vi "MFP assistant - Check leads connections.vi"(8 "Source":dbl[](array[numeric])=[1.0, 2.0, 3.0, 4.0, 5.0, 27.0, 28.0], 9 "Wait after changing source":dbl=5000.0, 10 "shunt resistor":dbl=100000.0 format="%#_13g", 11 "Excitation voltage":dbl=0.1) -> ()   [LabVIEW 2016]
uses:
  <userlib>/LevyLab/Lockin-Multichannel/Typedefs/AO-cluster.ctl
  <userlib>/LevyLab/Lockin-Multichannel/Typedefs/AO_Amp-array.ctl
  <userlib>/LevyLab/Lockin-Multichannel/Typedefs/AO_DC-array.ctl
  <userlib>/LevyLab/Lockin-Multichannel/Typedefs/AO_f-array.ctl
  <userlib>/LevyLab/Lockin-Multichannel/Typedefs/AO_phi-array.ctl
  <userlib>/LevyLab/Lockin-Multichannel/Typedefs/Function-array.ctl
  <userlib>/LevyLab/Lockin-Multichannel/Typedefs/Function-enum.ctl
panel:
  out "error out":errorcluster={"status"=TRUE, "code"=1000, "source"="Invoke Node in MFP assistant - Check leads connections.vi\n<APPEND>\nMethod Name: <b>Run VI</b>\n\nVI Path: <b>C:\\Program Files (x86)\\National Instruments\\LabVIEW 2016\\user.lib\\LevyLab\\Lockin-Multichannel\\Lockin-4461 -Patrick -State.vi</b>"}
  out "Drain":dbl=2.0
  out "Source":dbl=2.0
  out "2-T G":dbl=1.9062096105905893e-11 format="%#_6p"
  out "2-T G":dbl[][](array[numeric])=[[-1.000136832285521e-05, 1.2511313986118265e-10], [-4.380879926044356e-11, 1.9062096105905893e-11]] format="%#_4p"
  out "Drain":dbl[](array[numeric])=[1.0, 2.0]
  out "reference out":refnum<vi>
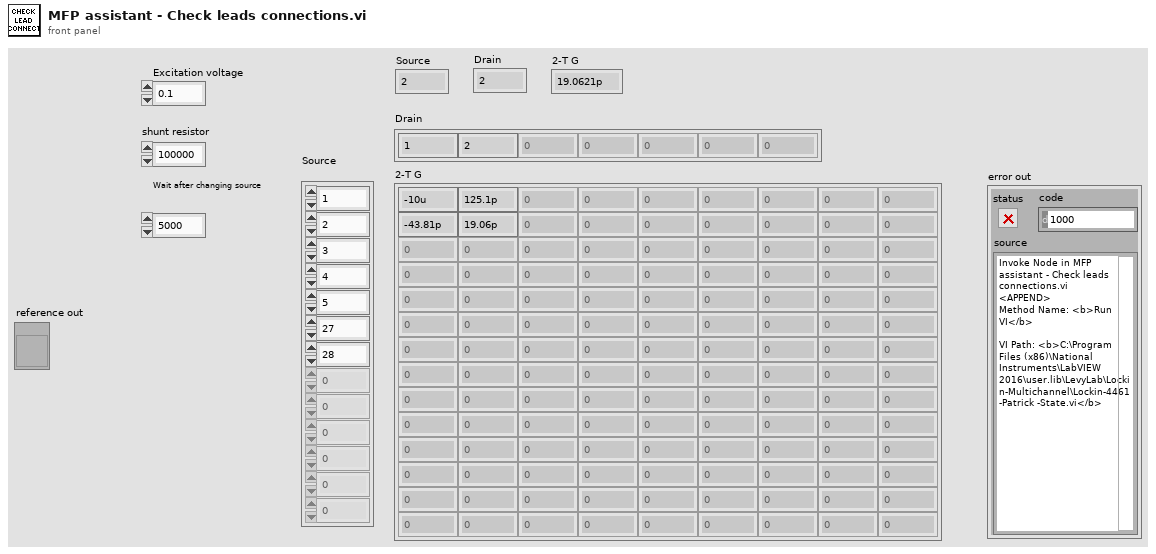
[diagram p1: front panel]
types:
  T1 = enum16{"Input array", "Manual", "All single-end", "All differential"}
  T2 = typedef "AO-cluster.ctl" = cluster{"AO amp (V)":T3, "AO DC (V)":T4, "AO f (Hz)":T5, "AO phi (deg)":T6, "function":T7}
  T3 = typedef "AO_Amp-array.ctl" = dbl[]
  T4 = typedef "AO_DC-array.ctl" = dbl[]
  T5 = typedef "AO_f-array.ctl" = dbl[]
  T6 = typedef "AO_phi-array.ctl" = dbl[]
  T7 = typedef "Function-array.ctl" = T8[]
  T8 = typedef "Function-enum.ctl" = enum16{"Sine Wave", "Triangle Wave", "Square Wave", "Sawtooth Wave"}
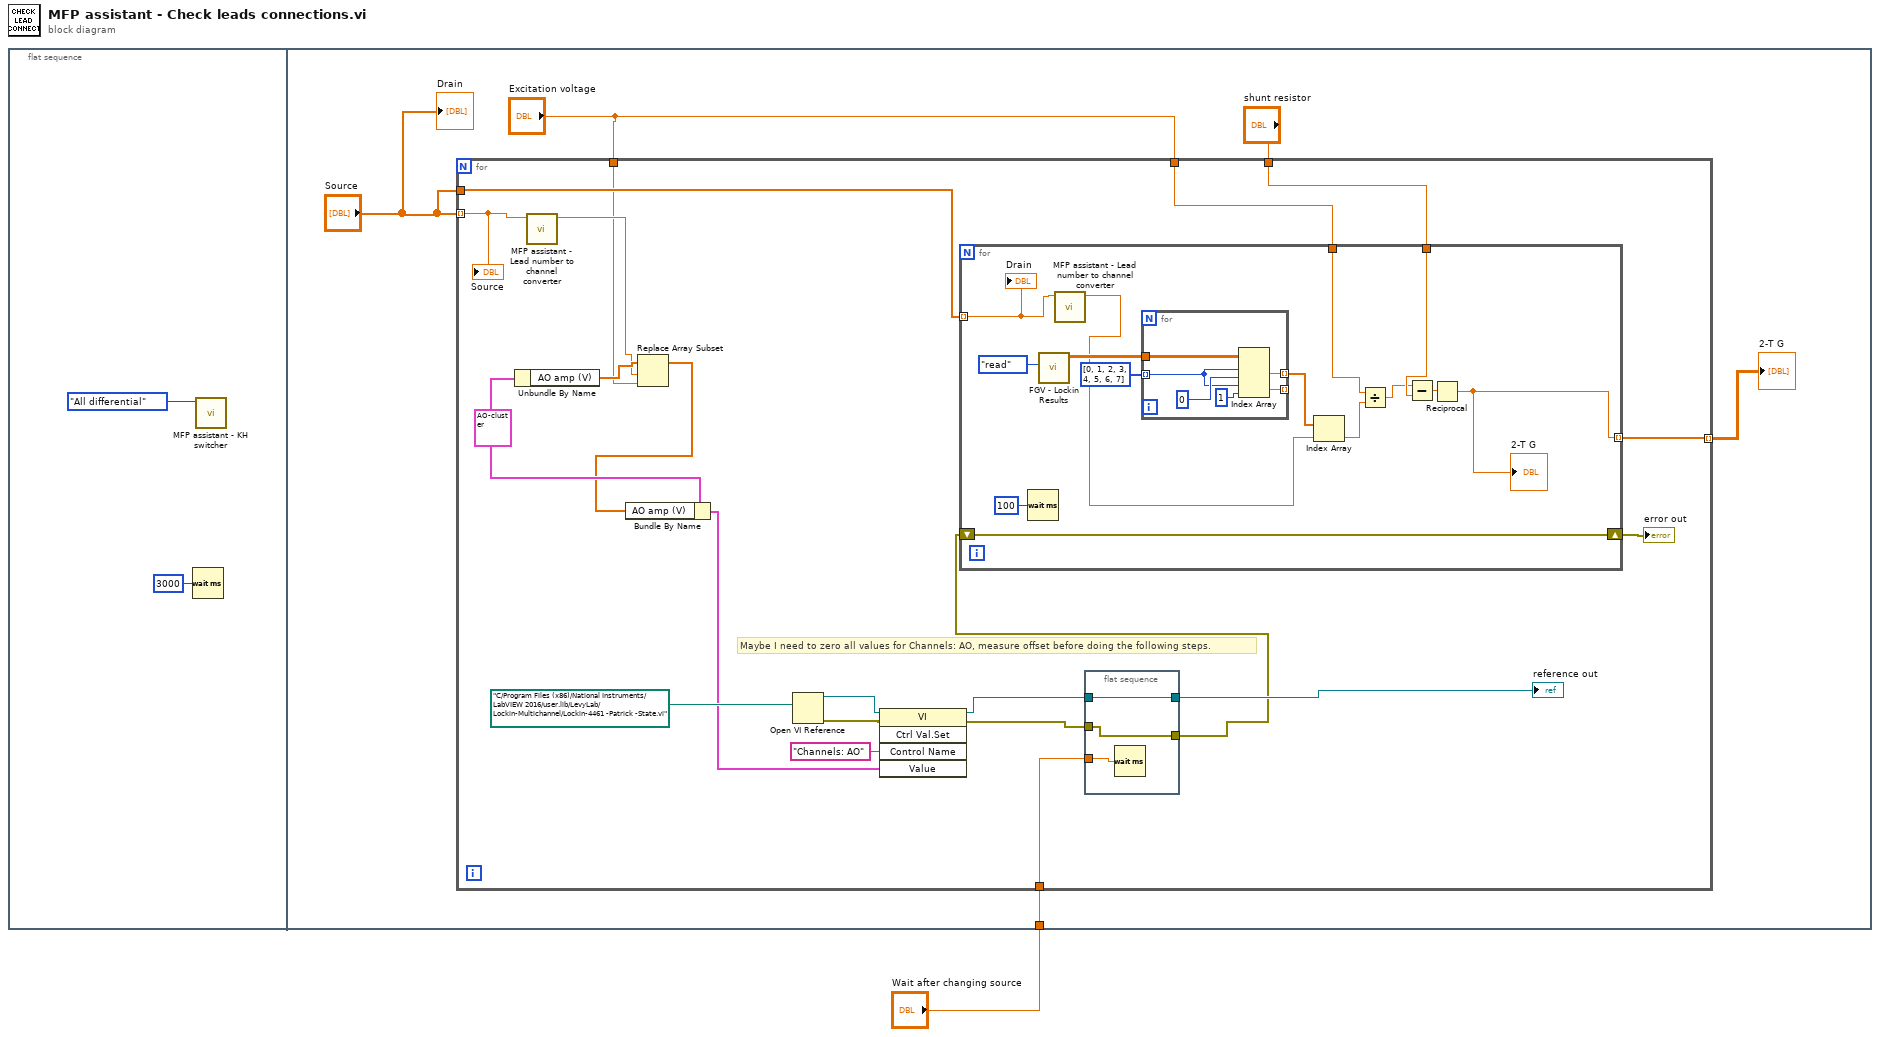
[diagram p0: block diagram]
diagram:
  n1 = flat-sequence {
    tunnel: "Wait after changing source" -> [w5]
    frame #0 {
      n2 = Wait (ms)(milliseconds to wait=u32 3000) -> ()  [unwired: 1 out]
      n3 = call "MFP assistant - KH switcher.vi"("KH setting"=T1."All differential") -> ()  [unwired: 11 in]
    }
    frame #1 {
      n4 = for {
        tunnel: "Source" -> [w28] mode=indexing
        tunnel: "Source" -> [w25]
        tunnel: [w17] -> w6 mode=indexing
        tunnel: "Excitation voltage" -> [w16]
        tunnel: "shunt resistor" -> [w15]
        tunnel: w5 -> [w10]
        tunnel: "Excitation voltage" -> [w9]
        w20 = T2 {"AO amp (V)"=[0.0, 0.0, 0.0, 0.0, 0.0, 0.0, 0.0, 0.0], "AO DC (V)"=[0.0, 0.0, 0.0, 0.0, 0.0, 0.0, 0.0, 0.0], "AO f (Hz)"=[13.0, 13.0, 13.0, 13.0, 13.0, 13.0, 13.0, 13.0], "AO phi (deg)"=[0.0, 0.0, 0.0, 0.0, 0.0, 0.0, 0.0, 0.0], "function"=[enum."Sine Wave", enum."Sine Wave", enum."Sine Wave", enum."Sine Wave", enum."Sine Wave", enum."Sine Wave", enum."Sine Wave", enum."Sine Wave"]} ("Initial settings for Channels: AO")
        # "Maybe I need to zero all values for Channels: AO, measure offset before doing the following steps."
        n5 = Unbundle By Name(w20) -> ("AO amp (V)"=w27:T3)
        n6 = call "MFP assistant - Lead number to channel converter.vi"("Lead number"=w28) -> ("Channel number (0, 1, 2,...)"=w26:dbl)  [unwired: 10 in]
        n7 = Replace Array Subset(array=w27, new element=w9, index=w26) -> (w19:T3)
        n8 = Bundle By Name(cluster=w20, "AO amp (V)"=w19) -> (w18:T2)
        n9 = Open VI Reference(vi path=path "C:/Program Files (x86)/National Instruments/LabVIEW 2016/user.lib/LevyLab/Lockin-Multichannel/Lockin-4461 -Patrick -State.vi") -> (vi reference=w23:refnum<vi>, error out=w22:errorcluster)  [unwired: 5 in]
        n10 = invoke class="VI" method="Ctrl Val.Set"(reference=w23, error in=w22, "Control Name"="Channels: AO", "Value"=w18) -> (reference out=w13:refnum<vi>, error out=w12:errorcluster)  [unwired: 1 in, 3 out]
        "reference out" <- w13
        n11 = for {
          tunnel: w25 -> [w34] mode=indexing
          tunnel: [w38] -> w17 mode=indexing
          tunnel: w16 -> [w37]
          tunnel: w15 -> [w41]
          shift-right: [w35] -> w14
          shift-left: w11 -> [w35]
          n12 = Wait (ms)(milliseconds to wait=u32 100) -> ()  [unwired: 1 out]
          n13 = call <userlib>:"FGV - Lockin Results.vi"("Function"=enum16{"write", "read"}."read") -> ("Input Signals"=w43:dbl[][])  [unwired: 5 in, 1 out]
          n14 = call "MFP assistant - Lead number to channel converter.vi"("Lead number"=w34) -> ("Channel number (0, 1, 2,...)"=w33:dbl)  [unwired: 10 in]
          n15 = for {
            tunnel: w43 -> [w48]
            tunnel: i32[] [0, 1, 2, 3, 4, 5, 6, 7] ("Lockins") -> [w49] mode=indexing
            tunnel: [w46] -> w42 mode=indexing
            tunnel: [w47] -> _ mode=indexing
            n16 = Index Array(array=w48, index (row) #1=w49, index (col) #1=0 ("disabled index (col)"), index (row) #2=w49, index (col) #2=1 ("disabled index (col)")) -> (element #1=w46:dbl, element #2=w47:dbl)
          }
          n17 = Index Array(array=w42, index=w33) -> (element=w36:dbl)
          n18 = Divide(x=w37, y=w36) -> (x/y=w40:dbl)
          n19 = Subtract(x=w40, y=w41) -> (x-y=w39:dbl)
          n20 = Reciprocal(x=w39) -> (1/x=w38:dbl)
          "2-T G" <- w38
          "Drain" <- w34
        }
        "error out" <- w14
        n21 = flat-sequence {
          tunnel: w13 -> [w31]
          tunnel: [w31] -> _
          tunnel: w12 -> [w30]
          tunnel: [w30] -> w11
          tunnel: w10 -> [w29]
          frame #0 {
            n22 = Wait (ms)(milliseconds to wait=w29) -> ()  [unwired: 1 out]
          }
        }
        "Source" <- w28
      }
      "2-T G" <- w6
      "Drain" <- "Source"
    }
  }
